vi "ep_Time Interpolation.vi"(7 "reset? (F)":bool, 8 "error in (no error)":errorcluster, 9 "samples per cycle":u16, 10 "triggers per cycle":u8, 11 "trigger positions [s]":dbl[](array[numeric])) -> (0 "error out":errorcluster, 3 "time index":dbl[](array[numeric]), 4 "last position [s]":dbl)   [LabVIEW 2013, in "NI_EP_Power Measurement.lvlib"]
uses:
  <vilib>/addons/Electrical Power/Power Measurement/NI_EP_Power Measurement.lvlib
  <vilib>/Analysis/1siggen.llb/Ramp Pattern by Samples.vi
  <vilib>/Analysis/2dsp.llb/Decimate (continuous, DBL).vi
  <vilib>/Analysis/NI_AALBase.lvlib
  <vilib>/Analysis/NI_AALPro.lvlib
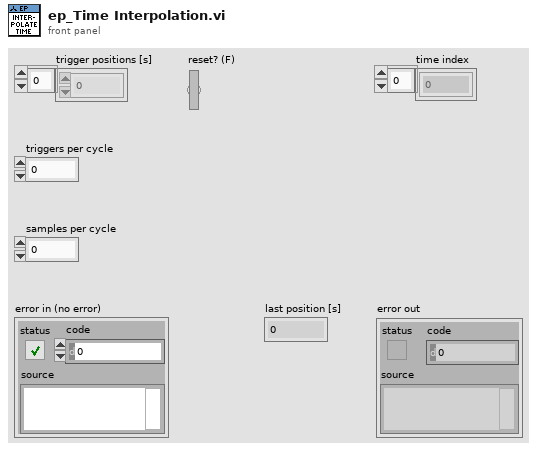
[diagram p1: front panel]
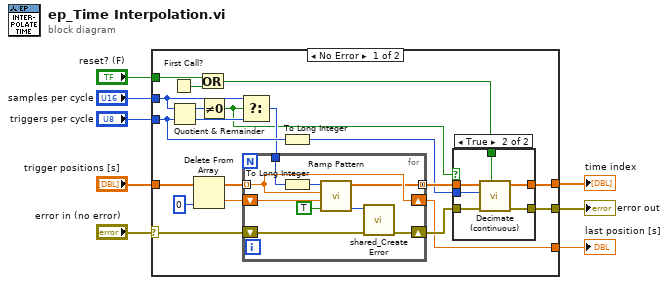
[diagram p0: block diagram]
diagram:
  n1 = case shown="No Error" "error in (no error)" {
    selector: "error in (no error)" -> [w24 w46]
    tunnel: [w26 _] -> w2
    tunnel: [w25 _] -> w1
    tunnel: [w23 w46] -> w7
    tunnel: "trigger positions [s]" -> [w20 _]
    tunnel: "reset? (F)" -> [w16 _]
    tunnel: "samples per cycle" -> [w13 _]
    tunnel: "triggers per cycle" -> [w12 _]
    frame No Error {
      n2 = First Call?() -> (First Call?: T/F=w22:bool)
      n3 = Quotient & Remainder(x=w13, y=w12) -> (x-y*floor(x/y)=w14:u16, floor(x/y)=w15:u16)
      n4 = Delete From Array(array=w20, index=0) -> (deleted portion=w18:dbl, array with subset deleted=w19:dbl[])  [unwired: 1 in]
      n5 = Or(x=w16, y=w22) -> (x .or. y?=w17:bool)
      n6 = Not Equal To 0?(x=w14) -> (x != 0?=w9:bool)
      n7 = Select(t=w13, s=w9, f=w15) -> (s? t:f=w11:u16)
      n8 = for {
        tunnel: w19 -> [w43] mode=indexing
        shift-right: [w43] -> w26
        shift-left: w18 -> [w45]
        shift-right: [w39] -> w27
        shift-left: w24 -> [w40]
        tunnel: [w42] -> w28 mode=concatenating
        tunnel: w11 -> [w37]
        n9 = To Long Integer(number=w37) -> (32bit integer=w41:i32)
        n10 = call-poly <vilib>:"Ramp Pattern.vi"("exclude end?"=TRUE, "start"=w45, "end"=w43, "samples"=w41) -> ("error"=w38:i32, "Ramp Pattern"=w42:dbl[])  [unwired: 6 in]
        n11 = call <vilib>:"shared_Create Error.vi"("error in (no error)"=w40, "error code (0)"=w38) -> ("error out"=w39:errorcluster)  [unwired: 9 in]
      }
      n12 = To Long Integer(number=w12) -> (32bit integer=w10:i32)
      n13 = case shown="True" w9 {
        tunnel: w10 -> [_ w34]
        tunnel: w28 -> [w30 w36]
        tunnel: w17 -> [_ w35]
        tunnel: w27 -> [w29 w33]
        tunnel: [w29 w32] -> w23
        tunnel: [w30 w31] -> w25
        frame False {
        }
        frame True {
          n14 = call-poly <vilib>:"Decimate (continuous).vi"("reset"=w35, "error in (no error)"=w33, "decimating factor"=w34, "X"=w36) -> ("error out"=w32:errorcluster, "Decimated Array"=w31:dbl[])  [unwired: 6 in]
        }
      }
    }
    frame Error {
    }
  }
  "error out" <- w7
  "time index" <- w1
  "last position [s]" <- w2
